vi "SetGraphTypes.vi"(1 "GraphTypes":refnum<class "Graph.lvclass">[](array[class]), 5 "error in (no error)":errorcluster) -> (19 "error out":errorcluster)   [LabVIEW 2020, in "Graph.lvclass"]
uses:
  <resource>/Framework/Providers/Open_GDS/UML/Graph_class/Graph.lvclass
  <resource>/Framework/Providers/Open_GDS/UML/AbstractNode_class/AbstractNode.lvclass
  <resource>/Framework/Providers/Open_GDS/UML/AbstractEdge_class/AbstractEdge.lvclass
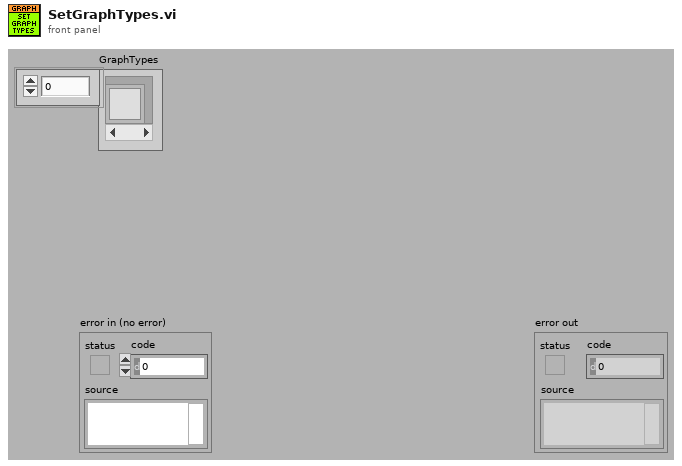
[diagram p1: front panel]
types:
  T1 = typedef "Graph.lvclass/ClassAttributes.ctl" = cluster{"NODE_PROT":refnum<class "AbstractNode.lvclass">[], "NodeNames":string[], "EDGE_PROT":refnum<class "AbstractEdge.lvclass">[], "EdgeNames":string[], "GraphTypes":refnum<class "Graph.lvclass">[], "GraphTypeNames":string[], "NodeTypes":refnum<class "AbstractNode.lvclass">[], "EdgeTypes":refnum<class "AbstractEdge.lvclass">[], "NodeTypeNames":string[], "EdgeTypeNames":string[]}
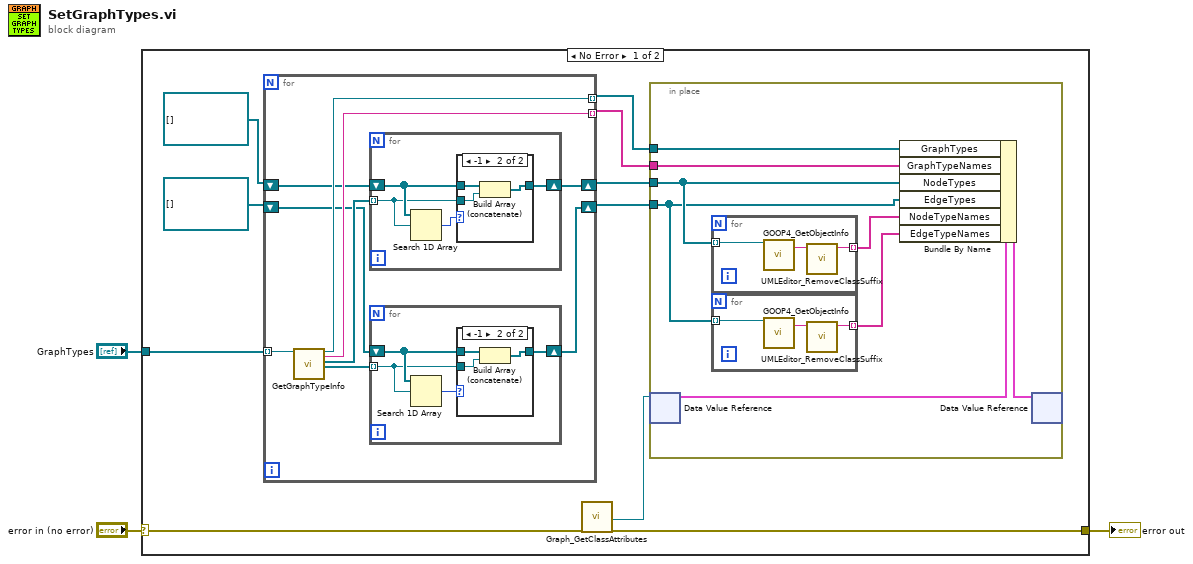
[diagram p0: block diagram]
diagram:
  n1 = case shown="No Error" "error in (no error)" {
    selector: "error in (no error)" -> [w5 w53]
    tunnel: [w4 w53] -> w2
    tunnel: "GraphTypes" -> [w12 _]
    frame No Error {
      n2 = for {
        tunnel: w12 -> [w36] mode=indexing
        tunnel: [w35] -> w11 mode=indexing
        tunnel: [w34] -> w10 mode=indexing
        shift-right: [w32] -> w9
        shift-left: refnum<class "AbstractNode.lvclass">[] [] -> [w33]
        shift-right: [w30] -> w6
        shift-left: refnum<class "AbstractEdge.lvclass">[] [] -> [w29]
        n3 = call-dynamic "GetGraphTypeInfo.vi"("reference in"=w36) -> ("reference out"=w34:refnum<class "Graph.lvclass">, "GraphTypeName"=w35:string, "NodeTypes"=w31:refnum<class "AbstractNode.lvclass">[], "EdgeTypes"=w28:refnum<class "AbstractEdge.lvclass">[])  [unwired: 13 in, 2 out]
        n4 = for {
          tunnel: w31 -> [w45] mode=indexing
          shift-right: [w48] -> w32
          shift-left: w33 -> [w47]
          n5 = Search 1D Array(1D array=w47, element=w45) -> (index of element=w46:i32)  [unwired: 1 in]
          n6 = case shown="-1" w46 {
            tunnel: [w49 w52] -> w48
            tunnel: w47 -> [w49 w51]
            tunnel: w45 -> [_ w50]
            frame 0, Default {
            }
            frame -1 {
              n7 = Build Array (concatenate)(w51, w50) -> (w52:refnum<class "AbstractNode.lvclass">[])
            }
          }
        }
        n8 = for {
          tunnel: w28 -> [w37] mode=indexing
          shift-right: [w40] -> w30
          shift-left: w29 -> [w39]
          n9 = Search 1D Array(1D array=w39, element=w37) -> (index of element=w38:i32)  [unwired: 1 in]
          n10 = case shown="-1" w38 {
            tunnel: [w41 w44] -> w40
            tunnel: w39 -> [w41 w43]
            tunnel: w37 -> [_ w42]
            frame 0, Default {
            }
            frame -1 {
              n11 = Build Array (concatenate)(w43, w42) -> (w44:refnum<class "AbstractEdge.lvclass">[])
            }
          }
        }
      }
      n12 = call <resource>:"Graph_GetClassAttributes.vi"("error in (no error)"=w5) -> ("Class attribute Reference"=w13:refnum<data-value>, "error out"=w4:errorcluster)  [unwired: 15 in, 2 out]
      n13 = in-place {
        in-place-border: w11 -> [w19]
        in-place-border: w10 -> [w18]
        in-place-border: w9 -> [w17]
        in-place-border: w6 -> [w15]
        n14 = in-place-dvr #1(w13) -> (w21:T1)  [unwired: 1 out]
        n15 = for {
          tunnel: w17 -> [w26] mode=indexing
          tunnel: [w25] -> w16 mode=indexing
          n16 = call <vilib>:"GOOP4_GetObjectInfo.vi"("ObjectIn"=w26) -> ("ObjectRuntimeClassName"=w27:string)  [unwired: 13 in, 5 out]
          n17 = call <resource>:"UMLEditor_RemoveClassSuffix.vi"("ObjectRuntimeClassName in"=w27) -> ("ObjectRuntimeClassName out"=w25:string)  [unwired: 10 in]
        }
        n18 = for {
          tunnel: w15 -> [w23] mode=indexing
          tunnel: [w22] -> w14 mode=indexing
          n19 = call <vilib>:"GOOP4_GetObjectInfo.vi"("ObjectIn"=w23) -> ("ObjectRuntimeClassName"=w24:string)  [unwired: 13 in, 5 out]
          n20 = call <resource>:"UMLEditor_RemoveClassSuffix.vi"("ObjectRuntimeClassName in"=w24) -> ("ObjectRuntimeClassName out"=w22:string)  [unwired: 10 in]
        }
        n21 = Bundle By Name(cluster=w21, "GraphTypes"=w18, "GraphTypeNames"=w19, "NodeTypes"=w17, "EdgeTypes"=w15, "NodeTypeNames"=w16, "EdgeTypeNames"=w14) -> (w20:T1)
        n22 = in-place-dvr #1(w20) -> ()  [unwired: 2 out]
      }
    }
    frame Error {
    }
  }
  "error out" <- w2
